vi "Add Exchanges.vi"(8 "error in (no error)":errorcluster caption="entrée d'erreur (pas d'erreur)", 10 "Exchange Added":refnum<class "Exchange.lvclass">, 11 "Exchanges en entrée":refnum<class "Exchanges.lvclass"> caption="DNL_LabVIEW Object in") -> (0 "error out":errorcluster caption="sortie d'erreur", 2 "created new?":bool, 3 "Exchanges en sortie":refnum<class "Exchanges.lvclass"> caption="DNL_LabVIEW Object out")   [LabVIEW 2012, in "Exchanges.lvclass"]
uses:
  Exchanges.lvclass
  Exchange/Exchange.lvclass
  <userlib>/_OpenG.lib/dictionary/dictionary.llb/Dictionary Key Value Pair Cluster__ogtk.ctl
  Exchanges.lvclass/Exchanges.ctl
  Exchange/Exchange.lvclass/Exchange.ctl
  <userlib>/_OpenG.lib/dictionary/dictionary.llb/Dictionary Update (by scalar value)__ogtk.vi
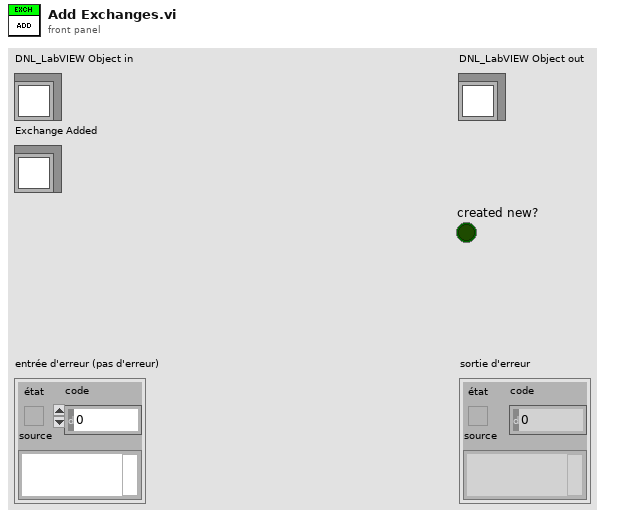
[diagram p1: front panel]
types:
  T1 = typedef "Dictionary Key Value Pair Cluster__ogtk.ctl" = cluster{"key":variant, "value":variant}
  T2 = typedef "Exchange Parameters.ctl" = cluster{"Date":timestamp, "Exchange Type":T3, "ISIN":string, "Label":string, "Price":dbl, "Qty":dbl, "Currency":T4, "Tax":dbl, "Comment":string, "PRU":dbl}
  T3 = typedef "Exchange.lvclass/Exchange Type Enum.ctl" = enum16{"ACHAT", "VENTE"}
  T4 = typedef "Currencies.ctl" = enum16{"Euro", "Dollar", "Yen", "RIM", "CHF"}
  T5 = typedef "Dictionary Object RefNum__ogtk.ctl" = refnum<k1>
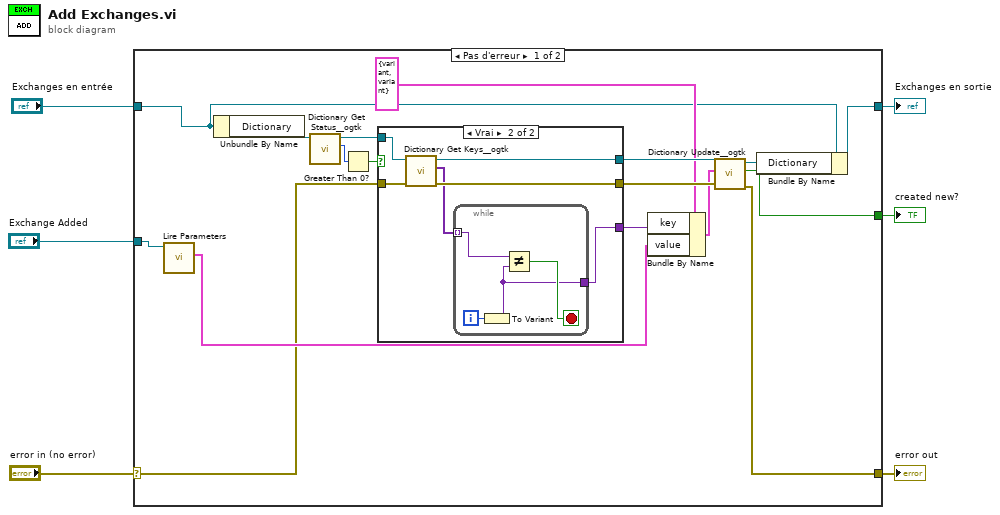
[diagram p0: block diagram]
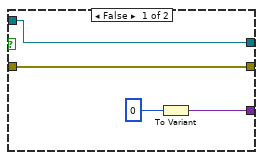
[diagram p2: hidden frame]
diagram:
  n1 = case shown="Pas d'erreur" "error in (no error)" {
    selector: "error in (no error)" -> [w9 w39]
    tunnel: [w10 w39] -> w5
    tunnel: [w8 w38] -> w3
    tunnel: "Exchanges en entrée" -> [w13 w38]
    tunnel: "Exchange Added" -> [w12 _]
    tunnel: [w7 _] -> w1
    frame No Error {
      n2 = call "Lire Parameters.vi"("Exchange en entrée"=w12) -> ("Parameters"=w11:T2)  [unwired: 9 in, 1 out]
      n3 = Unbundle By Name(w13) -> ("Dictionary"=w18:T5)
      n4 = call <userlib>:"Dictionary Get Status__ogtk.vi"("dictionary"=w18) -> ("size"=w17:i32, "dictionary out"=w16:T5)  [unwired: 8 in, 1 out]
      n5 = Greater Than 0?(x=w17) -> (x > 0?=w15:bool)
      n6 = case shown="Vrai" w15 {
        tunnel: [w24 w33] -> w22
        tunnel: w9 -> [w25 w32]
        tunnel: [w25 w31] -> w21
        tunnel: w16 -> [w24 w29]
        tunnel: [w26 w28] -> w14
        frame False {
          n7 = To Variant(anything=0 ("size")) -> (Variant=w26:variant)
        }
        frame True {
          n8 = call <userlib>:"Dictionary Get Keys__ogtk.vi"("error in (no error)"=w32, "dictionary"=w29) -> ("error out"=w31:errorcluster, "keys"=w30:variant[], "dictionary out"=w33:T5)  [unwired: 7 in]
          n9 = while {
            tunnel: w30 -> [w36] mode=indexing
            tunnel: [w34] -> w28
            i -> [w37]
            stop <- w35 stop-if-true
            n10 = To Variant(anything=w37) -> (Variant=w34:variant)
            n11 = Not Equal?(x=w36, y=w34) -> (x != y?=w35:bool)
          }
        }
      }
      n12 = Bundle By Name(cluster=T1 {"key"=variant, "value"=variant} ("key-value"), "key"=w14, "value"=w11) -> (w19:T1)
      n13 = call-poly <userlib>:"Dictionary Update__ogtk.vi"("error in (no error)"=w21, "key-value"=w19, "dictionary"=w22) -> ("error out"=w10:errorcluster, "created new?"=w7:bool, "dictionary out"=w23:T5)  [unwired: 6 in]
      n14 = Bundle By Name(cluster=w13, "Dictionary"=w23) -> (w8:refnum<class "Exchanges.lvclass">)
    }
    frame Error {
    }
  }
  "error out" <- w5
  "Exchanges en sortie" <- w3
  "created new?" <- w1
